vi "Read Single Point.vi"(8 "error in (no error)":errorcluster, 11 "VISA resource name":refnum<visa-resource-name>) -> (0 "error out":errorcluster, 2 "Measurement":dbl, 3 "VISA resource name out":refnum<visa-resource-name>)   [LabVIEW 2020, in "Library Instrument & Equipement.lvlib" / "Library Multimeter.lvlib" / "RIGOL DM3058.lvlib"]
doc: "Reads and returns a single measurement from the instrument."
uses:
  RIGOL DM3058.lvlib
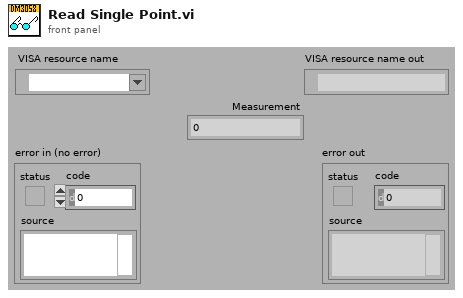
[diagram p1: front panel]
types:
  T1 = cluster{"DM Series Mode":u16, "Measurement Function":u16}
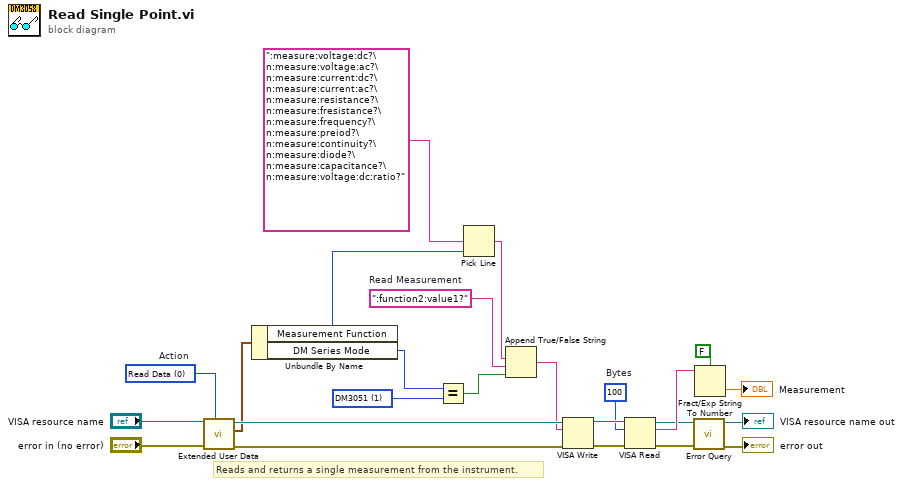
[diagram p0: block diagram]
diagram:
  w4 = u16 1 items=["DM3058", "DM3051", "DM3068", "DM3058E"] ("DM Series Mode")
  w15 = 0 items=["Read Data", "Write Data", "Clear Data", "Clear ALL Data"]  # Action
  w13 = ":function2:value1?"  # Read Measurement
  w22 = u32 100  # Bytes
  # "Reads and returns a single measurement from the instrument."
  n1 = call "Extended User Data.vi"("Action (1: Write Data)"=w15, "Error In (no error)"="error in (no error)", "VISA resource name in"="VISA resource name") -> ("Error Out"=w17:errorcluster, "User Data Out"=w2:T1, "VISA resource name out"=w16:refnum<visa-resource-name>)  [unwired: 1 in, 5 out]
  n2 = Unbundle By Name(w2) -> ("Measurement Function"=w12:u16, "DM Series Mode"=w1:u16)
  n3 = Equal?(x=w1, y=w4) -> (x = y?=w3:bool)
  n4 = Pick Line(multi-line string=":measure:voltage:dc?\n:measure:voltage:ac?\n:measure:current:dc?\n:measure:current:ac?\n:measure:resistance?\n:measure:fresistance?\n:measure:frequency?\n:measure:preiod?\n:measure:continuity?\n:measure:diode?\n:measure:capacitance?\n:measure:voltage:dc:ratio?", line index=w12) -> (output string=w10:string)  [unwired: 1 out]
  n5 = Append True/False String(1:w3, 2:w13, 3:w10) -> (0:w14:string)  [unwired: 1 out]
  n6 = VISA Write(VISA resource name=w16, write buffer=w14, error in (no error)=w17) -> (VISA resource name out=w23:refnum<visa-resource-name>, error out=w24:errorcluster)  [unwired: 1 out]
  n7 = VISA Read(VISA resource name=w23, byte count=w22, error in (no error)=w24) -> (VISA resource name out=w9:refnum<visa-resource-name>, read buffer=w20:string, error out=w8:errorcluster)  [unwired: 1 out]
  n8 = call "Error Query.vi"("error in (no error)"=w8, "VISA resource name"=w9) -> ("error out"=→"error out":errorcluster, "VISA resource name out"=→"VISA resource name out":refnum<visa-resource-name>)  [unwired: 8 out]
  n9 = Fract/Exp String To Number(use system decimal point (T)=FALSE, string=w20) -> (number=→"Measurement":dbl)  [unwired: 3 out]
